vi "myRIO_BRig_Host_formatData_getHeaders_dataLick.vi"() -> (3 "output_stringArray_dataLick":string[](array[string]))   [LabVIEW 2014]
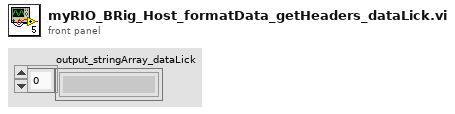
[diagram p1: front panel]
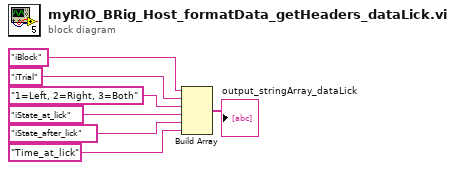
[diagram p0: block diagram]
diagram:
  n1 = Build Array("iBlock", "iTrial", "1=Left, 2=Right, 3=Both", "iState_at_lick", "iState_after_lick", "Time_at_lick") -> (→"output_stringArray_dataLick":string[])
